vi "BlinkM SetAddress.vi"(0 "Arduino Resource":T1={"VISA resource"="", "Board Type"=enum."Arduino Uno", "Connection Type"=enum."USB / Serial", "Bytes Per Packet (15)"=15}, 5 "Address":u8, 9 "New Address":u8, 11 "error in":errorcluster) -> (4 "Arduino Resource":T1={"VISA resource"="", "Board Type"=enum."Arduino Uno", "Connection Type"=enum."USB / Serial", "Bytes Per Packet (15)"=15}, 15 "error out":errorcluster)   [LabVIEW 2011, in "LabVIEW Interface for Arduino.lvlib"]
doc: "Assign a new I2C address to the specified BlinkM. Valid address must be between 1 and 127."
uses:
  LabVIEW Interface for Arduino.lvlib
  Private/Type Defs/Arduino Resource.ctl
  Private/Type Defs/Board Type.ctl
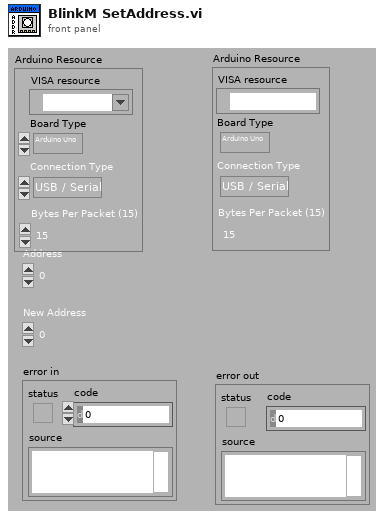
[diagram p1: front panel]
types:
  T1 = typedef "LabVIEW Interface for Arduino.lvlib/Arduino Resource.ctl" = cluster{"VISA resource":refnum<visa-resource-name>, "Board Type":T2, "Connection Type":enum8{"USB / Serial"}, "Bytes Per Packet (15)":u8}
  T2 = typedef "LabVIEW Interface for Arduino.lvlib/Board Type.ctl" = enum16{"Arduino Uno", "Dimuelanove w/Atmega 328", "Mega 2560", "Chipkit Uno32", "Chipkit Max32"}
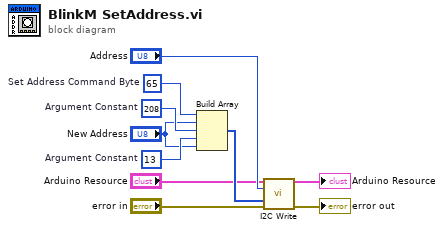
[diagram p0: block diagram]
diagram:
  w5 = u8 13  # Argument Constant
  w4 = u8 208  # Argument Constant
  w7 = u8 65  # Set Address Command Byte
  n1 = Build Array(w7, "New Address", w4, w5, "New Address") -> (w6:u8[])
  n2 = call "I2C Write.vi"("Arduino Resource"="Arduino Resource", "Address (0)"="Address", "I2C Data Bytes"=w6, "error in"="error in") -> ("Arduino Resource"=→"Arduino Resource":T1, "error out"=→"error out":errorcluster)  [unwired: 10 in]
